vi "PH_Beckhoff-16BB.declare Tags.vi"(4 "error in (no error)":errorcluster, 7 "Instance Name":string) -> (0 "error out":errorcluster, 1 "Racktype":string, 3 "Data in cluster":T1={"Default Values"={"Sonderklemmen Inputs"=[], "Analog Inputs"=[], "Analog Outputs"=[], "Digital Inputs"=[], "Digital Outputs"=[]}, "Description"="", "Hardware configured?"=TRUE, "Activate Change Manager?"=FALSE, "Difference to handle an analog input as change"=1})   [LabVIEW 2014, in "PH_Beckhoff-16BB.lvlib"]
doc: "This VI declares the tagnames and sets the scaling of the tags of this class."
uses:
  PH_Beckhoff-16BB.lvlib
  PH_Beckhoff/PH_Beckhoff.constructor Data in.ctl
  PH_Beckhoff/PH_Beckhoff.Values.ctl
  PH_Beckhoff/PH_Beckhoff.Sonderklemmen Inputs.ctl
  PH_Beckhoff/PH_Beckhoff.Analog Inputs.ctl
  PH_Beckhoff/PH_Beckhoff.Scaling Type.ctl
  PH_Beckhoff/PH_Beckhoff.Analog Outputs.ctl
  PH_Beckhoff/PH_Beckhoff.Digital Inputs.ctl
  PH_Beckhoff/PH_Beckhoff.Digital Outputs.ctl
  PH_Beckhoff/PH_Beckhoff.lvlib
  PH_Basics/PH_Common/PH_Common.lvlib
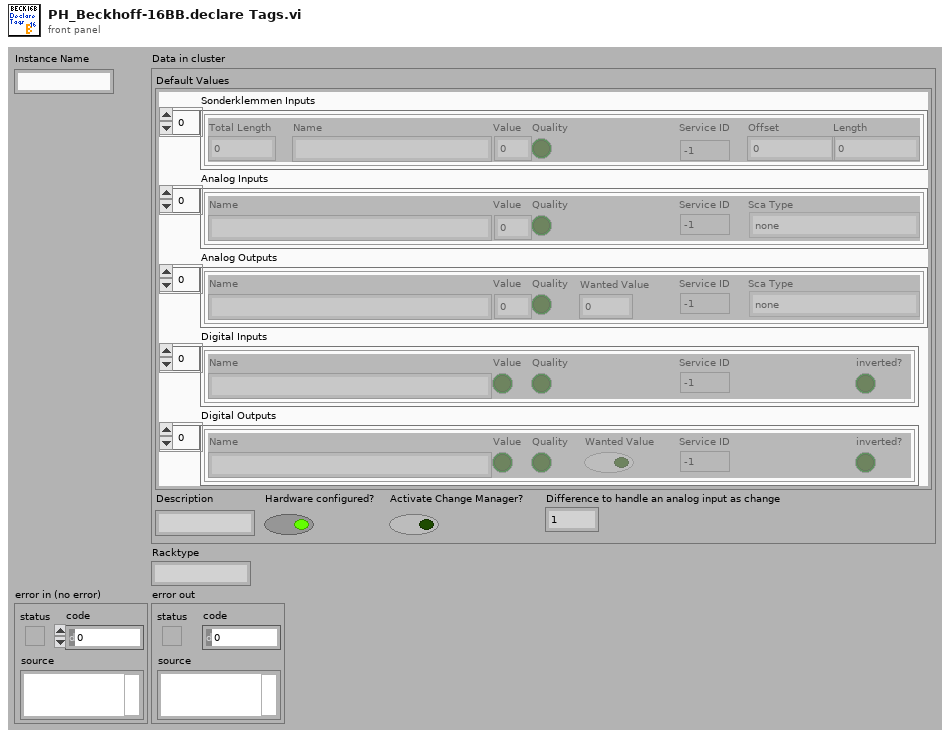
[diagram p1: front panel]
types:
  T1 = typedef "PH_Beckhoff.lvlib/PH_Beckhoff.constructor Data in.ctl" = cluster{"Default Values":T2, "Description":string, "Hardware configured?":bool, "Activate Change Manager?":bool, "Difference to handle an analog input as change":u32}
  T2 = typedef "PH_Beckhoff.lvlib/PH_Beckhoff.Values.ctl" = cluster{"Sonderklemmen Inputs":T3, "Analog Inputs":T4, "Analog Outputs":T6, "Digital Inputs":T7, "Digital Outputs":T8}
  T3 = typedef "PH_Beckhoff.lvlib/PH_Beckhoff.Sonderklemmen Inputs.ctl" = cluster{"Total Length":u32, "Name":string, "Value":u64, "Quality":bool, "Service ID":i32, "Offset":u32, "Length":u32}[]
  T4 = typedef "PH_Beckhoff.lvlib/PH_Beckhoff.Analog Inputs.ctl" = cluster{"Name":string, "Value":u32, "Quality":bool, "Service ID":i32, "Sca Type":T5}[]
  T5 = typedef "PH_Beckhoff.lvlib/PH_Beckhoff.Scaling Type.ctl" = enum16{"none", "0 ... 15 Bit -> 0 ... 5", "0 ... 15 Bit -> 0 ... 10", "0 ... 15 Bit -> 0 ... 25", "0 ... 15 Bit -> 4 ... 20", "0 ... 15 Bit -> 0 ... 1", "0 ... 15 Bit -> 0 ... 20000", "0 ... 15 Bit -> 0 ... 24000"}
  T6 = typedef "PH_Beckhoff.lvlib/PH_Beckhoff.Analog Outputs.ctl" = cluster{"Name":string, "Value":u32, "Quality":bool, "Wanted Value":u32, "Service ID":i32, "Sca Type":T5}[]
  T7 = typedef "PH_Beckhoff.lvlib/PH_Beckhoff.Digital Inputs.ctl" = cluster{"Name":string, "Value":bool, "Quality":bool, "Service ID":i32, "inverted?":bool}[]
  T8 = typedef "PH_Beckhoff.lvlib/PH_Beckhoff.Digital Outputs.ctl" = cluster{"Name":string, "Value":bool, "Quality":bool, "Wanted Value":bool, "Service ID":i32, "inverted?":bool}[]
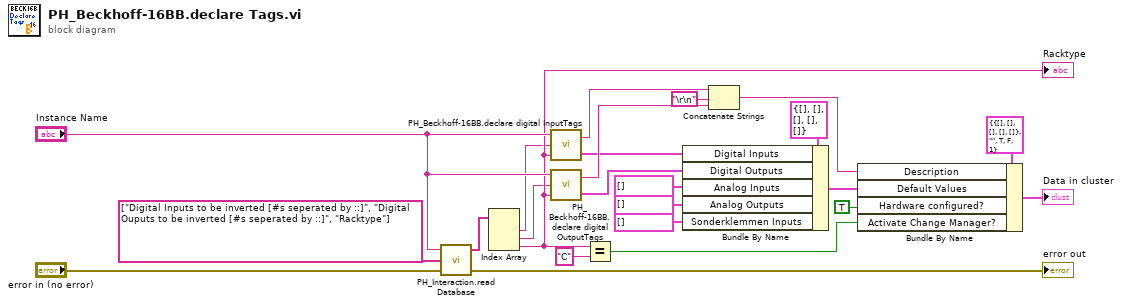
[diagram p0: block diagram]
diagram:
  n1 = call "PH_Interaction.read Database.vi"("error in (no error)"="error in (no error)", "Strings to search for"=string[] ["Digital Inputs to be inverted [#s seperated by ::]", "Digital Ouputs to be inverted [#s seperated by ::]", "Racktype"] ("Strings to search for in"), "DB Entry to read"="Instance Name") -> ("error out"=→"error out":errorcluster, "Values"=w5:string[])  [unwired: 1 in]
  n2 = Index Array(array=w5) -> (element #1=w3:string, element #2=w2:string, element #3=w4:string)  [unwired: 3 in]
  "Racktype" <- w4
  n3 = call "PH_Beckhoff-16BB.declare digital InputTags.vi"("Racktype"=w4, "Digital Inputs to be inverted [#s separated by ::]"=w3, "Instance Name"="Instance Name") -> ("Digital Inputs"=w9:T7, "Description"=w18:string)
  n4 = call "PH_Beckhoff-16BB.declare digital OutputTags.vi"("Racktype"=w4, "Digital Outputs to be inverted [#s separated by ::]"=w2, "Instance Name"="Instance Name") -> ("Digital Outputs"=w13:T8, "Description"=w17:string)
  n5 = Equal?(x=w4, y="C") -> (x = y?=w10:bool)
  n6 = Bundle By Name(cluster=T2 {"Sonderklemmen Inputs"=[], "Analog Inputs"=[], "Analog Outputs"=[], "Digital Inputs"=[], "Digital Outputs"=[]} ("Dummy Default Values"), "Digital Inputs"=w9, "Digital Outputs"=w13, "Analog Inputs"=T4 [], "Analog Outputs"=T6 [], "Sonderklemmen Inputs"=T3 []) -> (w20:T2)
  n7 = Concatenate Strings(w18, "\r\n", w17) -> (w16:string)
  n8 = Bundle By Name(cluster=T1 {"Default Values"={"Sonderklemmen Inputs"=[], "Analog Inputs"=[], "Analog Outputs"=[], "Digital Inputs"=[], "Digital Outputs"=[]}, "Description"="", "Hardware configured?"=TRUE, "Activate Change Manager?"=FALSE, "Difference to handle an analog input as change"=1} ("Dummy data in cluster"), "Description"=w16, "Default Values"=w20, "Hardware configured?"=TRUE, "Activate Change Manager?"=w10) -> (→"Data in cluster":T1)
